vi "Example Callback - DetectionCycleEnded Callback.vi"(4 "DetectionCycleEnded":refnum<user-event>, 5 "Event Data":cluster{"sender":refnum<k24>}, 6 "Control Ref":refnum<k24>, 7 "Event Common Data":T1) -> ()   [LabVIEW 2013]
uses:
  C:/tf/play/labview/Tinkerforge.dll
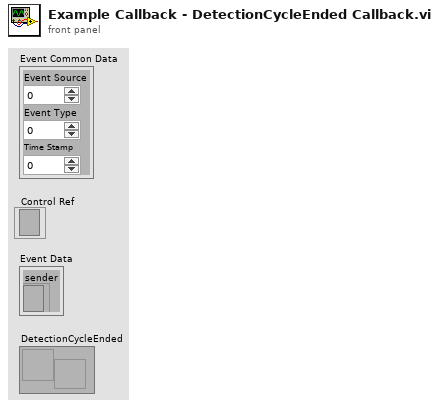
[diagram p1: front panel]
types:
  T1 = cluster{"Event Source":i32, "Event Type":u32, "Time Stamp":u32}
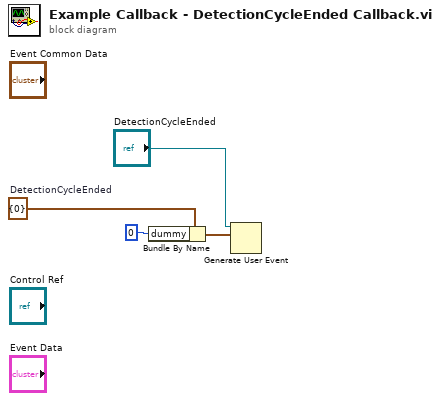
[diagram p0: block diagram]
diagram:
  w4 = cluster{"dummy":u8} {"dummy"=0}  # DetectionCycleEnded
  n1 = Bundle By Name(cluster=w4, "dummy"=u8 0) -> (w2:cluster{"dummy":u8})
  n2 = Generate User Event(user event="DetectionCycleEnded", event data cluster=w2) -> ()  [unwired: 2 in, 2 out]
